vi "RichToFlatnidaqmx_grpc_CreateCIFreqChanRequest.vi"(5 "OutputClusterType":T1, 11 "InputCluster":T6) -> (3 "OutputCluster":T1)   [LabVIEW 2021, in "NI DAQmx_server.lvlib"]
uses:
  NI DAQmx_server.lvlib
  nidaqmx_grpc_CreateCIFreqChanRequest.ctl
  nidevice_grpc_Session_session/nidevice_grpc_Session_session.lvclass
  nidaqmx_grpc_CreateCIFreqChanRequest_units_enum/nidaqmx_grpc_CreateCIFreqChanRequest_units_enum.lvclass
  nidaqmx_grpc_CreateCIFreqChanRequest_edge_enum/nidaqmx_grpc_CreateCIFreqChanRequest_edge_enum.lvclass
  nidaqmx_grpc_CreateCIFreqChanRequest_meas_method_enum/nidaqmx_grpc_CreateCIFreqChanRequest_meas_method_enum.lvclass
  nidevice_grpc_Session.ctl
  nidaqmx_grpc_CreateCIFreqChanRequest_Flat.ctl
  nidevice_grpc_Session_Flat.ctl
  nidaqmx_grpc_FrequencyUnits3.ctl
  nidaqmx_grpc_Edge1.ctl
  nidaqmx_grpc_CounterFrequencyMethod.ctl
  nidevice_grpc_Session_session/nidevice_grpc_Session_session.lvclass/nidevice_grpc_Session_session.ctl
  nidaqmx_grpc_CreateCIFreqChanRequest_units_enum/nidaqmx_grpc_CreateCIFreqChanRequest_units_enum.lvclass/nidaqmx_grpc_CreateCIFreqChanRequest_units_enum.ctl
  nidaqmx_grpc_CreateCIFreqChanRequest_edge_enum/nidaqmx_grpc_CreateCIFreqChanRequest_edge_enum.lvclass/nidaqmx_grpc_CreateCIFreqChanRequest_edge_enum.ctl
  nidaqmx_grpc_CreateCIFreqChanRequest_meas_method_enum/nidaqmx_grpc_CreateCIFreqChanRequest_meas_method_enum.lvclass/nidaqmx_grpc_CreateCIFreqChanRequest_meas_method_enum.ctl
  nidevice_grpc_Session_session/Getname.vi
  nidevice_grpc_Session_session/Getid.vi
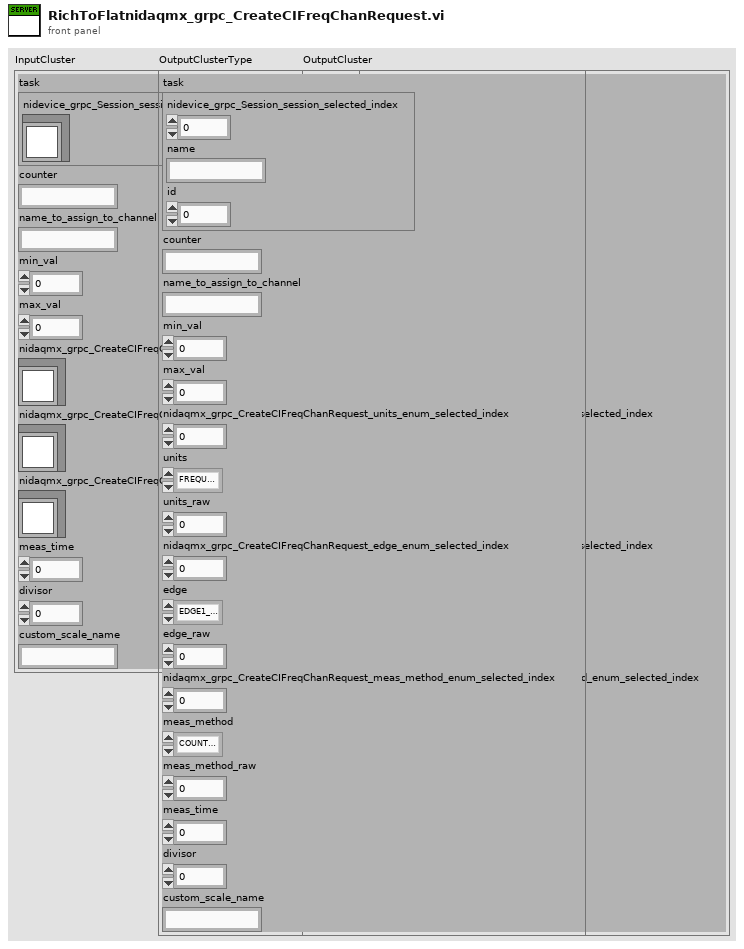
[diagram p1: front panel]
types:
  T1 = typedef "NI DAQmx_server.lvlib/nidaqmx_grpc_CreateCIFreqChanRequest_Flat.ctl" = cluster{"task":T2, "counter":string, "name_to_assign_to_channel":string, "min_val":dbl, "max_val":dbl, "nidaqmx_grpc_CreateCIFreqChanRequest_units_enum_selected_index":i32, "units":T3, "units_raw":i32, "nidaqmx_grpc_CreateCIFreqChanRequest_edge_enum_selected_index":i32, "edge":T4, "edge_raw":i32, "nidaqmx_grpc_CreateCIFreqChanRequest_meas_method_enum_selected_index":i32, "meas_method":T5, "meas_method_raw":i32, "meas_time":dbl, "divisor":u32, "custom_scale_name":string}
  T2 = typedef "NI DAQmx_server.lvlib/nidevice_grpc_Session_Flat.ctl" = cluster{"nidevice_grpc_Session_session_selected_index":i32, "name":string, "id":u32}
  T3 = typedef "NI DAQmx_server.lvlib/nidaqmx_grpc_FrequencyUnits3.ctl" = enum32{"FREQUENCY_UNITS3_UNSPECIFIED", "FREQUENCY_UNITS3_HZ", "FREQUENCY_UNITS3_TICKS", "FREQUENCY_UNITS3_FROM_CUSTOM_SCALE"}
  T4 = typedef "NI DAQmx_server.lvlib/nidaqmx_grpc_Edge1.ctl" = enum32{"EDGE1_UNSPECIFIED", "EDGE1_RISING", "EDGE1_FALLING"}
  T5 = typedef "NI DAQmx_server.lvlib/nidaqmx_grpc_CounterFrequencyMethod.ctl" = enum32{"COUNTER_FREQUENCY_METHOD_UNSPECIFIED", "COUNTER_FREQUENCY_METHOD_LOW_FREQ_1_CTR", "COUNTER_FREQUENCY_METHOD_HIGH_FREQ_2_CTR", "COUNTER_FREQUENCY_METHOD_LARGE_RNG_2_CTR", "COUNTER_FREQUENCY_METHOD_DYN_AVG"}
  T6 = typedef "NI DAQmx_server.lvlib/nidaqmx_grpc_CreateCIFreqChanRequest.ctl" = cluster{"task":T7, "counter":string, "name_to_assign_to_channel":string, "min_val":dbl, "max_val":dbl, "nidaqmx_grpc_CreateCIFreqChanRequest_units_enum":refnum<class "nidaqmx_grpc_CreateCIFreqChanRequest_units_enum.lvclass">, "nidaqmx_grpc_CreateCIFreqChanRequest_edge_enum":refnum<class "nidaqmx_grpc_CreateCIFreqChanRequest_edge_enum.lvclass">, "nidaqmx_grpc_CreateCIFreqChanRequest_meas_method_enum":refnum<class "nidaqmx_grpc_CreateCIFreqChanRequest_meas_method_enum.lvclass">, "meas_time":dbl, "divisor":u32, "custom_scale_name":string}
  T7 = typedef "NI DAQmx_server.lvlib/nidevice_grpc_Session.ctl" = cluster{"nidevice_grpc_Session_session":refnum<class "nidevice_grpc_Session_session.lvclass">}
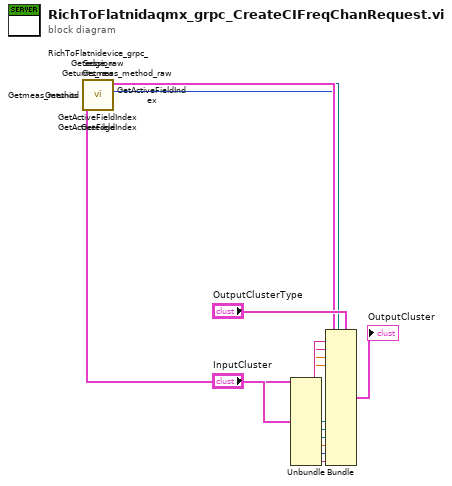
[diagram p0: block diagram]
diagram:
  n1 = Unbundle "Unbundle"("InputCluster") -> ("task"=w21:T7, "counter"=w19:string, "name_to_assign_to_channel"=w18:string, "min_val"=w17:dbl, "max_val"=w16:dbl, "nidaqmx_grpc_CreateCIFreqChanRequest_units_enum"=w15:refnum<class "nidaqmx_grpc_CreateCIFreqChanRequest_units_enum.lvclass">, "nidaqmx_grpc_CreateCIFreqChanRequest_edge_enum"=w11:refnum<class "nidaqmx_grpc_CreateCIFreqChanRequest_edge_enum.lvclass">, "nidaqmx_grpc_CreateCIFreqChanRequest_meas_method_enum"=w7:refnum<class "nidaqmx_grpc_CreateCIFreqChanRequest_meas_method_enum.lvclass">, "meas_time"=w3:dbl, "divisor"=w2:u32, "custom_scale_name"=w1:string)
  n2 = call "Getmeas_method_raw.vi"("OneOfTemplate in"=w7) -> ("Get_Val"=w4:i32)  [unwired: 8 in, 2 out]
  n3 = call "Getmeas_method.vi"("OneOfTemplate in"=w7) -> ("Get_Val"=w5:T5)  [unwired: 8 in, 2 out]
  n4 = call "GetActiveFieldIndex.vi"("OneOfTemplate in"=w7) -> ("Active Field Index"=w6:i32)  [unwired: 8 in, 2 out]
  n5 = call "Getedge_raw.vi"("OneOfTemplate in"=w11) -> ("Get_Val"=w8:i32)  [unwired: 8 in, 2 out]
  n6 = call "Getedge.vi"("OneOfTemplate in"=w11) -> ("Get_Val"=w9:T4)  [unwired: 8 in, 2 out]
  n7 = call "GetActiveFieldIndex.vi"("OneOfTemplate in"=w11) -> ("Active Field Index"=w10:i32)  [unwired: 8 in, 2 out]
  n8 = call "Getunits_raw.vi"("OneOfTemplate in"=w15) -> ("Get_Val"=w12:i32)  [unwired: 8 in, 2 out]
  n9 = call "Getunits.vi"("OneOfTemplate in"=w15) -> ("Get_Val"=w13:T3)  [unwired: 8 in, 2 out]
  n10 = call "GetActiveFieldIndex.vi"("OneOfTemplate in"=w15) -> ("Active Field Index"=w14:i32)  [unwired: 8 in, 2 out]
  n11 = call "RichToFlatnidevice_grpc_Session.vi"("InputCluster"=w21) -> ("OutputCluster"=w20:T2)  [unwired: 10 in]
  n12 = Bundle "Bundle"(cluster="OutputClusterType", "task"=w20, "counter"=w19, "name_to_assign_to_channel"=w18, "min_val"=w17, "max_val"=w16, "nidaqmx_grpc_CreateCIFreqChanRequest_units_enum_selected_index"=w14, "units"=w13, "units_raw"=w12, "nidaqmx_grpc_CreateCIFreqChanRequest_edge_enum_selected_index"=w10, "edge"=w9, "edge_raw"=w8, "nidaqmx_grpc_CreateCIFreqChanRequest_meas_method_enum_selected_index"=w6, "meas_method"=w5, "meas_method_raw"=w4, "meas_time"=w3, "divisor"=w2, "custom_scale_name"=w1) -> (→"OutputCluster":T1)
